vi "POI Gen Engine.vi"(9 "Function":T1) -> (2 "empty?":bool)   [LabVIEW 2013]
uses:
  Typedefs/Duplicate POI function enum.ctl
  <vilib>/vision/Image Controls.llb/IMAQ Image.ctl
  Typedefs/ROI ID Enum.ctl
  Globals/gl_ROI Entry UI globals.vi
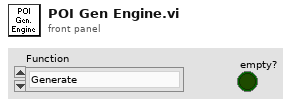
[diagram p1: front panel]
types:
  T1 = typedef "Duplicate POI function enum.ctl" = enum16{"Generate", "Adjust number of POI", "Clear register"}
  T2 = typedef "IMAQ Image.ctl" = refnum<image>
  T3 = typedef "ROI entry screen ctrl refs cluster.ctl" = cluster{"Done button":refnum<vi>, "Imaging button":refnum<vi>, "Acquisition button":refnum<vi>, "POI dwell time (us)":refnum<vi>, "Scan dwell time per pixel (us)":refnum<vi>, "# of planes":refnum<vi>, "Zoom":refnum<vi>, "Equal size":refnum<vi>, "Channel":refnum<vi>, "Image Display":refnum<vi>, "Z-Plane Selector":refnum<vi>, "Number of lines left":refnum<vi>, "Z-stack folder path":refnum<vi>, "POI Density":refnum<vi>, "Arb Plane Entry":refnum<vi>, "Whole plane":refnum<vi>, "Clear Last":refnum<vi>, "Clear All":refnum<vi>, "Trial Length (sec)":refnum<vi>, "Palette Type":refnum<vi>, "Intensity slider":refnum<vi>, "# POI":refnum<vi>, "Max Z Proj":refnum<vi>, "Zplane ind":refnum<vi>, "Wavelength (nm)":refnum<vi>, "Number of Trials":refnum<vi>, "Funct stim.trig.enable":refnum<vi>, "Funct stim.trig.delay (s)":refnum<vi>, "Line Mode":refnum<vi>, "Step size (µm)":refnum<vi>, "ROI move mode":refnum<vi>, "Cool-down time (s)":refnum<vi>, "Enable cool-down time":refnum<vi>, "Motor Z ind. (um)":refnum<vi>, "AOL Z ind. (um)":refnum<vi>}
  T4 = cluster{"Global Rectangle":i32[], "Contours":cluster{"Contour Type":u32, "ROI Type":u32, "Points":i32[]}[]}
  T5 = typedef "ROI ID Enum.ctl" = enum16{"Point", "MiniScan", "Comp. MiniScan", "Rectangle", "Comp. volume", "Arb. plane point"}
  T6 = cluster{"Pos. X":i32, "Pos. Y":i32, "Radius":i32, "Core Area":i32}[]
  T7 = typedef "ROI spec.ctl" = cluster{"Coordinates":i32[], "Zoom":dbl, "ROI Enum":T5, "ZplaneIndex":i32}
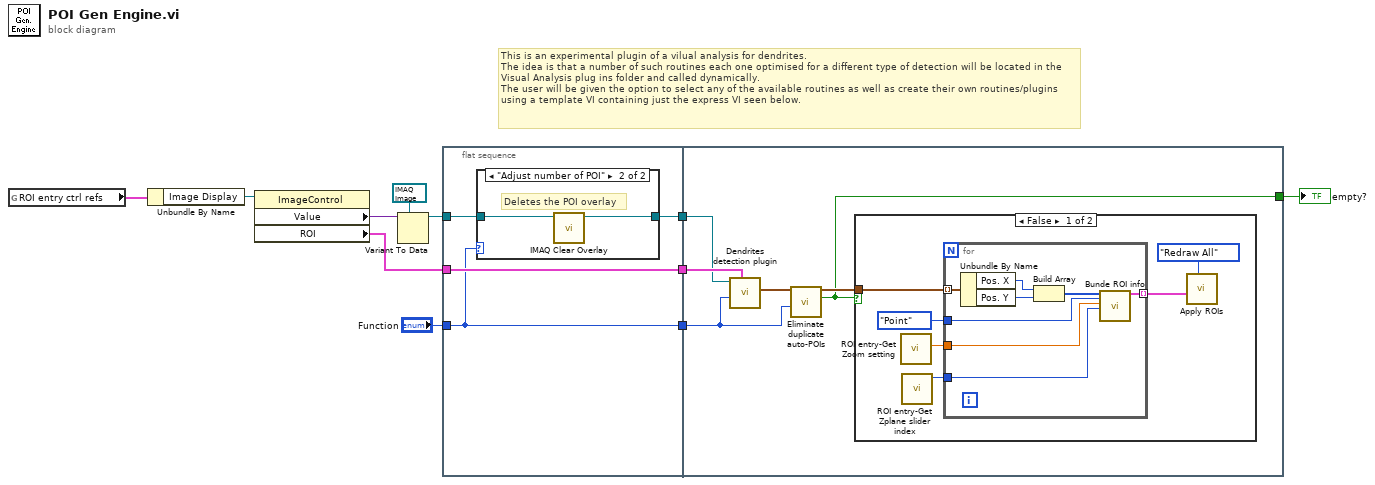
[diagram p0: block diagram]
diagram:
  # "This is an experimental plugin of a vilual analysis for dendrites.\nThe idea is that a number of such routines each one optimised for a different type of detection will be located in the Visual Analysis plug ins folder and called dynamically.\nThe user will be given the option to select any of the available routines as well as create their own routines/plugins using a template VI containing just the express VI seen below."
  n1 = global read "gl_ROI Entry UI globals.vi" "ROI entry ctrl refs"() -> (w1:T3)
  n2 = Unbundle By Name(w1) -> ("Image Display"=w6:refnum<vi>)
  n3 = property class="ImageControl"(reference=w6) -> ("Value"=w5:variant, "ROI"=w2:T4)  [unwired: 1 in, 2 out]
  n4 = Variant To Data(type=T2 refnum ("Image ref in"), Variant=w5) -> (data=w3:T2)  [unwired: 1 in, 1 out]
  n5 = flat-sequence {
    tunnel: "Function" -> [w12]
    tunnel: [w12] -> w11
    tunnel: w2 -> [w15]
    tunnel: [w15] -> w10
    tunnel: [w13] -> w9
    tunnel: w3 -> [w14]
    tunnel: w11 -> [w20]
    tunnel: w10 -> [w22]
    tunnel: w9 -> [w21]
    tunnel: [w19] -> w8
    frame #0 {
      n6 = case shown="\"Adjust number of POI\"" w12 {
        tunnel: w14 -> [w16 w18]
        tunnel: [w16 w17] -> w13
        frame "Generate", Default {
        }
        frame "Adjust number of POI" {
          # "Deletes the POI overlay"
          n7 = call "IMAQ Clear Overlay"("Image"=w18) -> ("Image Out"=w17:T2)  [unwired: 9 in, 1 out]
        }
      }
    }
    frame #1 {
      n8 = call "Dendrites detection plugin.vi"("ROI"=w22, "Function"=w20, "16 bit image in"=w21) -> ("Circles Data"=w23:T6)  [unwired: 5 in, 3 out]
      n9 = call "Eliminate duplicate auto-POIs.vi"("Function"=w20, "Circles Data in"=w23) -> ("empty?"=w19:bool, "Circles Data out"=w24:T6)  [unwired: 8 in]
      n10 = case shown="False" w19 {
        tunnel: w24 -> [w30 _]
        frame False {
          n11 = call "ROI entry-Get Zoom setting.vi"() -> ("Zoom Value"=w28:dbl)  [unwired: 9 in, 2 out]
          n12 = call "ROI entry-Get Zplane slider index.vi"() -> ("Z-plane slider's index (zero-based)"=w25:i32)  [unwired: 10 in, 1 out]
          n13 = for {
            tunnel: w30 -> [w36] mode=indexing
            tunnel: w28 -> [w34]
            tunnel: [w33] -> w29 mode=indexing
            tunnel: ROI_ID_Enum."Point" ("ROI Enum") -> [w32]
            tunnel: w25 -> [w31]
            n14 = Unbundle By Name(w36) -> ("Pos. X"=w37:i32, "Pos. Y"=w38:i32)
            n15 = Build Array(w37, w38) -> (w35:i32[])
            n16 = call "Bunde ROI info.vi"("ROI Coordinates"=w35, "ROI Enum"=w32, "Zoom"=w34, "ZplaneIndex"=w31) -> ("ROI Info"=w33:T7)  [unwired: 15 in]
          }
          n17 = call "Apply ROIs.vi"("Mode (Redraw All)"=enum16{"Redraw All", "Draw Last"}."Redraw All", "ROIs Info []"=w29) -> ()  [unwired: 6 in, 4 out]
        }
        frame True {
        }
      }
    }
  }
  "empty?" <- w8
